vi "DelayR_ext.vi"(6 "DelayR reg old":T1, 7 "T  ms (0 curr)":u32, 8 "R":bool, 9 "DelayOff (0)":u32, 10 "DelayOn (0)":u32, 11 "In":bool) -> (2 "t ms":u32, 3 "Out":bool, 4 "DelayR reg":T1)   [LabVIEW 2019, in "Timers.lvlib"]
uses:
  Timers.lvlib
  Logik/Logik.lvlib
  Trigers/Triggers.lvlib
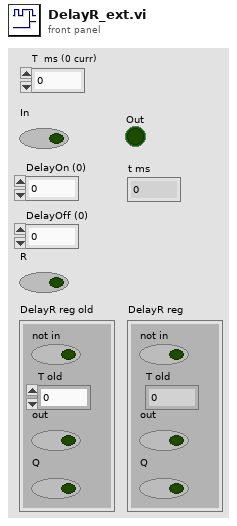
[diagram p1: front panel]
types:
  T1 = cluster{"not in":bool, "T old":u32, "out":bool, "Q":bool}
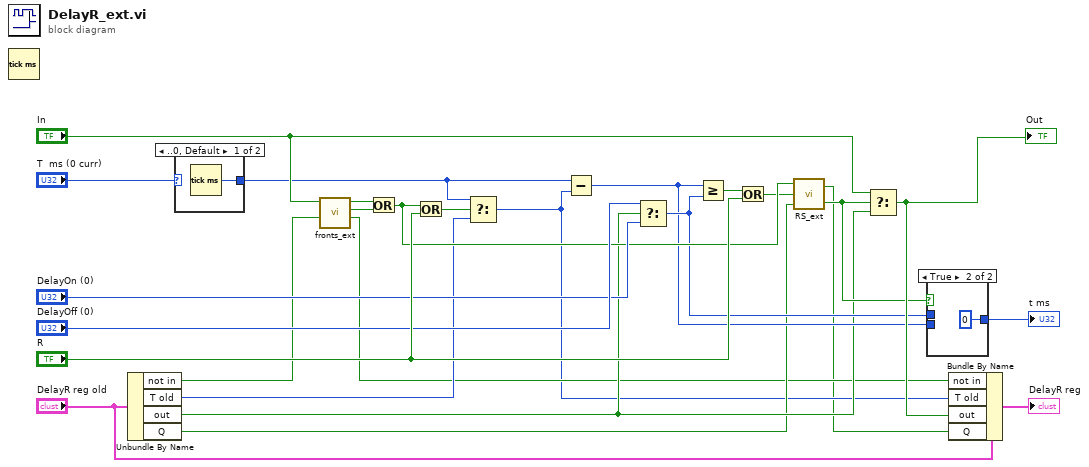
[diagram p0: block diagram]
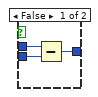
[diagram p3: hidden frame]
diagram:
  n1 = Tick Count (ms)() -> ()  [unwired: 1 out]
  n2 = Unbundle By Name("DelayR reg old") -> ("not in"=w8:bool, "T old"=w7:u32, "out"=w6:bool, "Q"=w5:bool)
  n3 = case shown="..0, Default" "T  ms (0 curr)" {
    selector: "T  ms (0 curr)" -> [_ w28]
    tunnel: [w27 w28] -> w1
    frame ..0, Default {
      n4 = Tick Count (ms)() -> (millisecond timer value=w27:u32)
    }
    frame 1.. {
    }
  }
  n5 = call "fronts_ext.vi"("not in old"=w8, "in"="In") -> ("not in"=w4:bool, "fall"=w16:bool, "raise"=w17:bool)  [unwired: 3 in]
  n6 = Or(x=w17, y=w16) -> (x .or. y?=w14:bool)
  n7 = Or(x=w14, y="R") -> (x .or. y?=w15:bool)
  n8 = Select(t=w1, s=w15, f=w7) -> (s? t:f=w3:u32)
  n9 = Subtract(x=w1, y=w3) -> (x-y=w9:u32)
  n10 = Select(t="DelayOff (0)", s=w6, f="DelayOn (0)") -> (s? t:f=w10:u32)
  n11 = Greater Or Equal?(x=w9, y=w10) -> (x >= y?=w13:bool)
  n12 = Or(x=w13, y="R") -> (x .or. y?=w12:bool)
  n13 = call "RS_ext.vi"("Q old"=w5, "R"=w12, "S"=w14) -> ("~Q"=w11:bool, "Q"=w2:bool)
  n14 = Select(t="In", s=w11, f=w6) -> (s? t:f=w18:bool)
  "Out" <- w18
  n15 = case shown="True" w11 {
    tunnel: w10 -> [w31 _]
    tunnel: w9 -> [w30 _]
    tunnel: [w29 u32 0] -> w25
    frame False {
      n16 = Subtract(x=w31, y=w30) -> (x-y=w29:u32)
    }
    frame True {
    }
  }
  "t ms" <- w25
  n17 = Bundle By Name(cluster="DelayR reg old", "not in"=w4, "T old"=w3, "out"=w18, "Q"=w2) -> (→"DelayR reg":T1)
